vi "TTL_XOR_with_IO_inv_config.vi"(10 "IO inversion config.":u8, 11 "TTL port(s) config to fire":u8) -> (2 "OFF config.":u32, 3 "ON config.":u32)   [LabVIEW 2018, in "TTL IO.lvlib"]
uses:
  TTL IO.lvlib
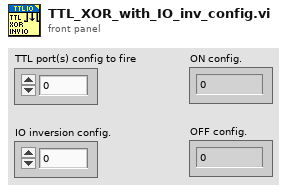
[diagram p1: front panel]
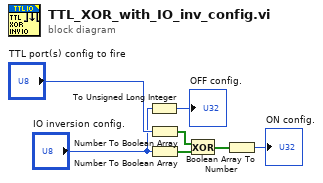
[diagram p0: block diagram]
diagram:
  n1 = To Unsigned Long Integer(number="IO inversion config.") -> (unsigned 32bit integer=→"OFF config.":u32)
  n2 = Number To Boolean Array(number="TTL port(s) config to fire") -> (Boolean array=w5:bool[])
  n3 = Number To Boolean Array(number="IO inversion config.") -> (Boolean array=w4:bool[])
  n4 = Exclusive Or(1:w4, 2:w5) -> (0:w3:bool[])
  n5 = Boolean Array To Number(Boolean array=w3) -> (number=→"ON config.":u32)
